vi "pulse_generator_data_v3.vi"(4 "Vapor Inlet Temp [C]":dbl, 5 "Power":dbl, 6 "PG Data":waveform(dbl)[](array[waveform]), 7 "Offsets":T4={"PG Abs"=0.0, "PG Pitot dP"=11500.0, "W1-4 dP "=0.0, "W1-7 dP"=11500.0, "W1-7 Fast dP"=0.0, "TS W1 Abs P"=11500.0, "TS W7 Abs P"=0.0, "Vapor Line Pitot dP"=0.0}, 8 "Session Start Time":timestamp) -> (0 "Pulse Generator Charts":T2, 1 "Diode Charts":T1, 2 "Measurements":T3={"PG Abs Pressure"=119484.80284900061, "Vapor Temperature"=19.805676371442082, "Liquid Temperature"=19.52526901660894, "Tinlet"=121.24568157832624, "Tsectwo"=119.96937909943745, "TS Abs Pressure W1"=121.24568157832624, "TS Abs Pressure W7"=119.96937909943745, "W1-4 dP[Pa]"=19.52526901660894, "W1-7 dP[Pa]"=119.96937909943745, "W1-7 dP[Pa] Fast"=119.96937909943745, "PG Venturi dP [Pa]"=119.96937909943745, "Vapor Line Pitot dP [Pa]"=119.96937909943745, "Tsecthree"=19.191961040039615, "Toutlet"=19.148186089917207, "TS Ext"=18.97439824494449, "Vapor Sat Pressure"=121.24568157832624, "Liquid Sat Pressure"=119.96937909943745, "PG Mass Flow Rate"=nan, "Vapor Line Mass Flow"=119.96937909943745}, 3 "PG Data - Queue":dbl[][](array[numeric]))   [LabVIEW 2017]
uses:
  Sensor Translation/sensor_translation.lvlib
  Sensor Translation/Pressure Transducers/Omega/omega_px209_060a5v.vi
  Sensor Translation/Pressure Transducers/Rosemont/rosemont_3051C_d_1_a_2_2_a_1_a.vi
  Sensor Translation/Pressure Transducers/Omega/omega_px409_2-5ddui.vi
  diode_charts.ctl
  <vilib>/Waveform/WDTOps.llb/WDT Get Waveform Time Array DBL.vi
  pulse_generator_data_controls.ctl
  pulse_generator_data.ctl
  pulse_generator_data_charts.ctl
panel:
  out "Main Diode":dbl[](array[numeric])
  # "Test Section"
  # "Pulse Gen"
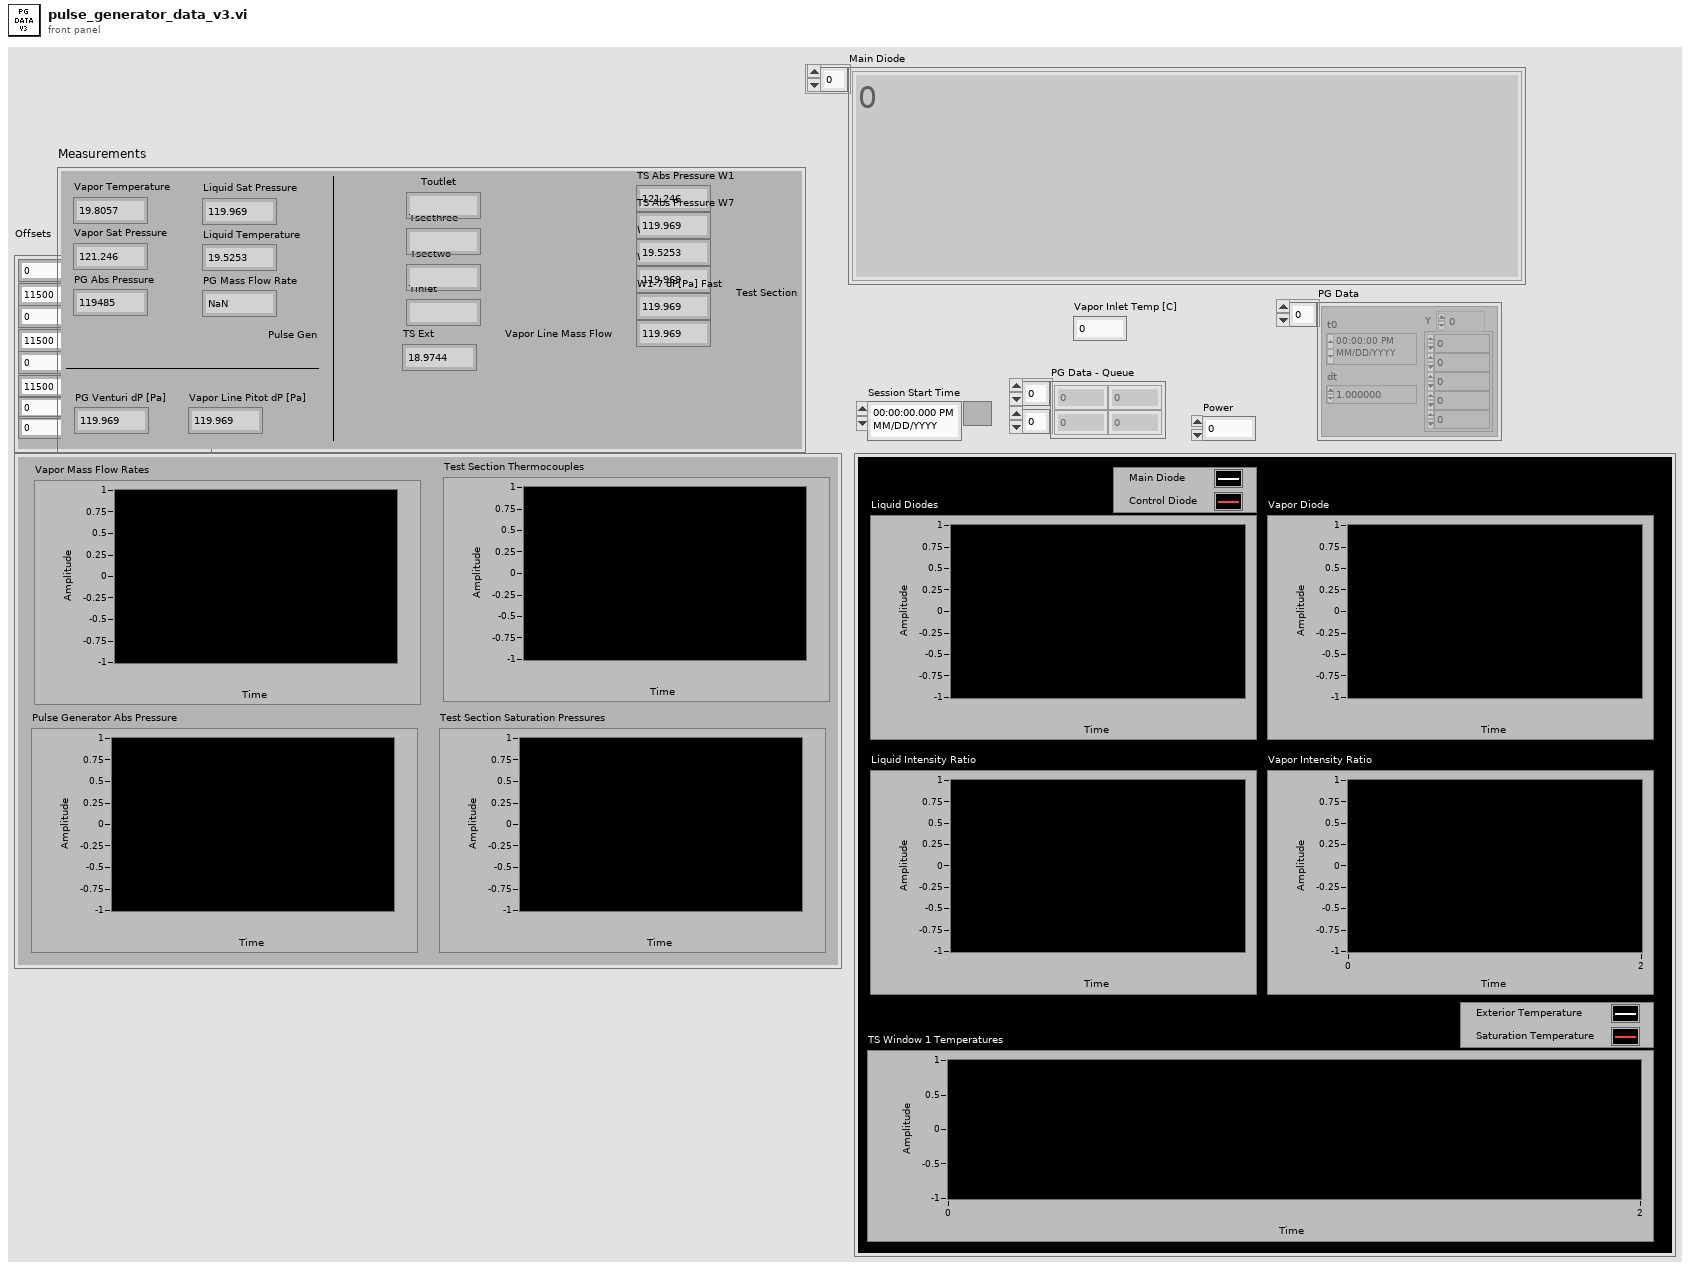
[diagram p1: front panel]
types:
  T1 = typedef "diode_charts.ctl" = cluster{"Liquid Diodes":cluster{dbl, dbl}, "Liquid Intensity Ratio":dbl, "Vapor Diode":cluster{dbl, dbl}, "Vapor Intensity Ratio":dbl, "TS Window 1 Temperatures":cluster{"Average":dbl, "T Sat [C]":dbl}}
  T2 = typedef "pulse_generator_data_charts.ctl" = cluster{"Vapor Mass Flow Rates":cluster{"max value":dbl, "max value":dbl}, "Test Section Thermocouples":cluster{"[0]":dbl, "[1]":dbl, "[2]":dbl, "[3]":dbl, "[4]":dbl}, "Pulse Generator Abs Pressure":dbl[], "Test Section Saturation Pressures":cluster{"max value":dbl, "max value":dbl}}
  T3 = typedef "pulse_generator_data.ctl" = cluster{"PG Abs Pressure":dbl, "Vapor Temperature":dbl, "Liquid Temperature":dbl, "Tinlet":dbl, "Tsectwo":dbl, "TS Abs Pressure W1":dbl, "TS Abs Pressure W7":dbl, "W1-4 dP[Pa]":dbl, "W1-7 dP[Pa]":dbl, "W1-7 dP[Pa] Fast":dbl, "PG Venturi dP [Pa]":dbl, "Vapor Line Pitot dP [Pa]":dbl, "Tsecthree":dbl, "Toutlet":dbl, "TS Ext":dbl, "Vapor Sat Pressure":dbl, "Liquid Sat Pressure":dbl, "PG Mass Flow Rate":dbl, "Vapor Line Mass Flow":dbl}
  T4 = typedef "pulse_generator_data_controls.ctl" = cluster{"PG Abs":dbl, "PG Pitot dP":dbl, "W1-4 dP ":dbl, "W1-7 dP":dbl, "W1-7 Fast dP":dbl, "TS W1 Abs P":dbl, "TS W7 Abs P":dbl, "Vapor Line Pitot dP":dbl}
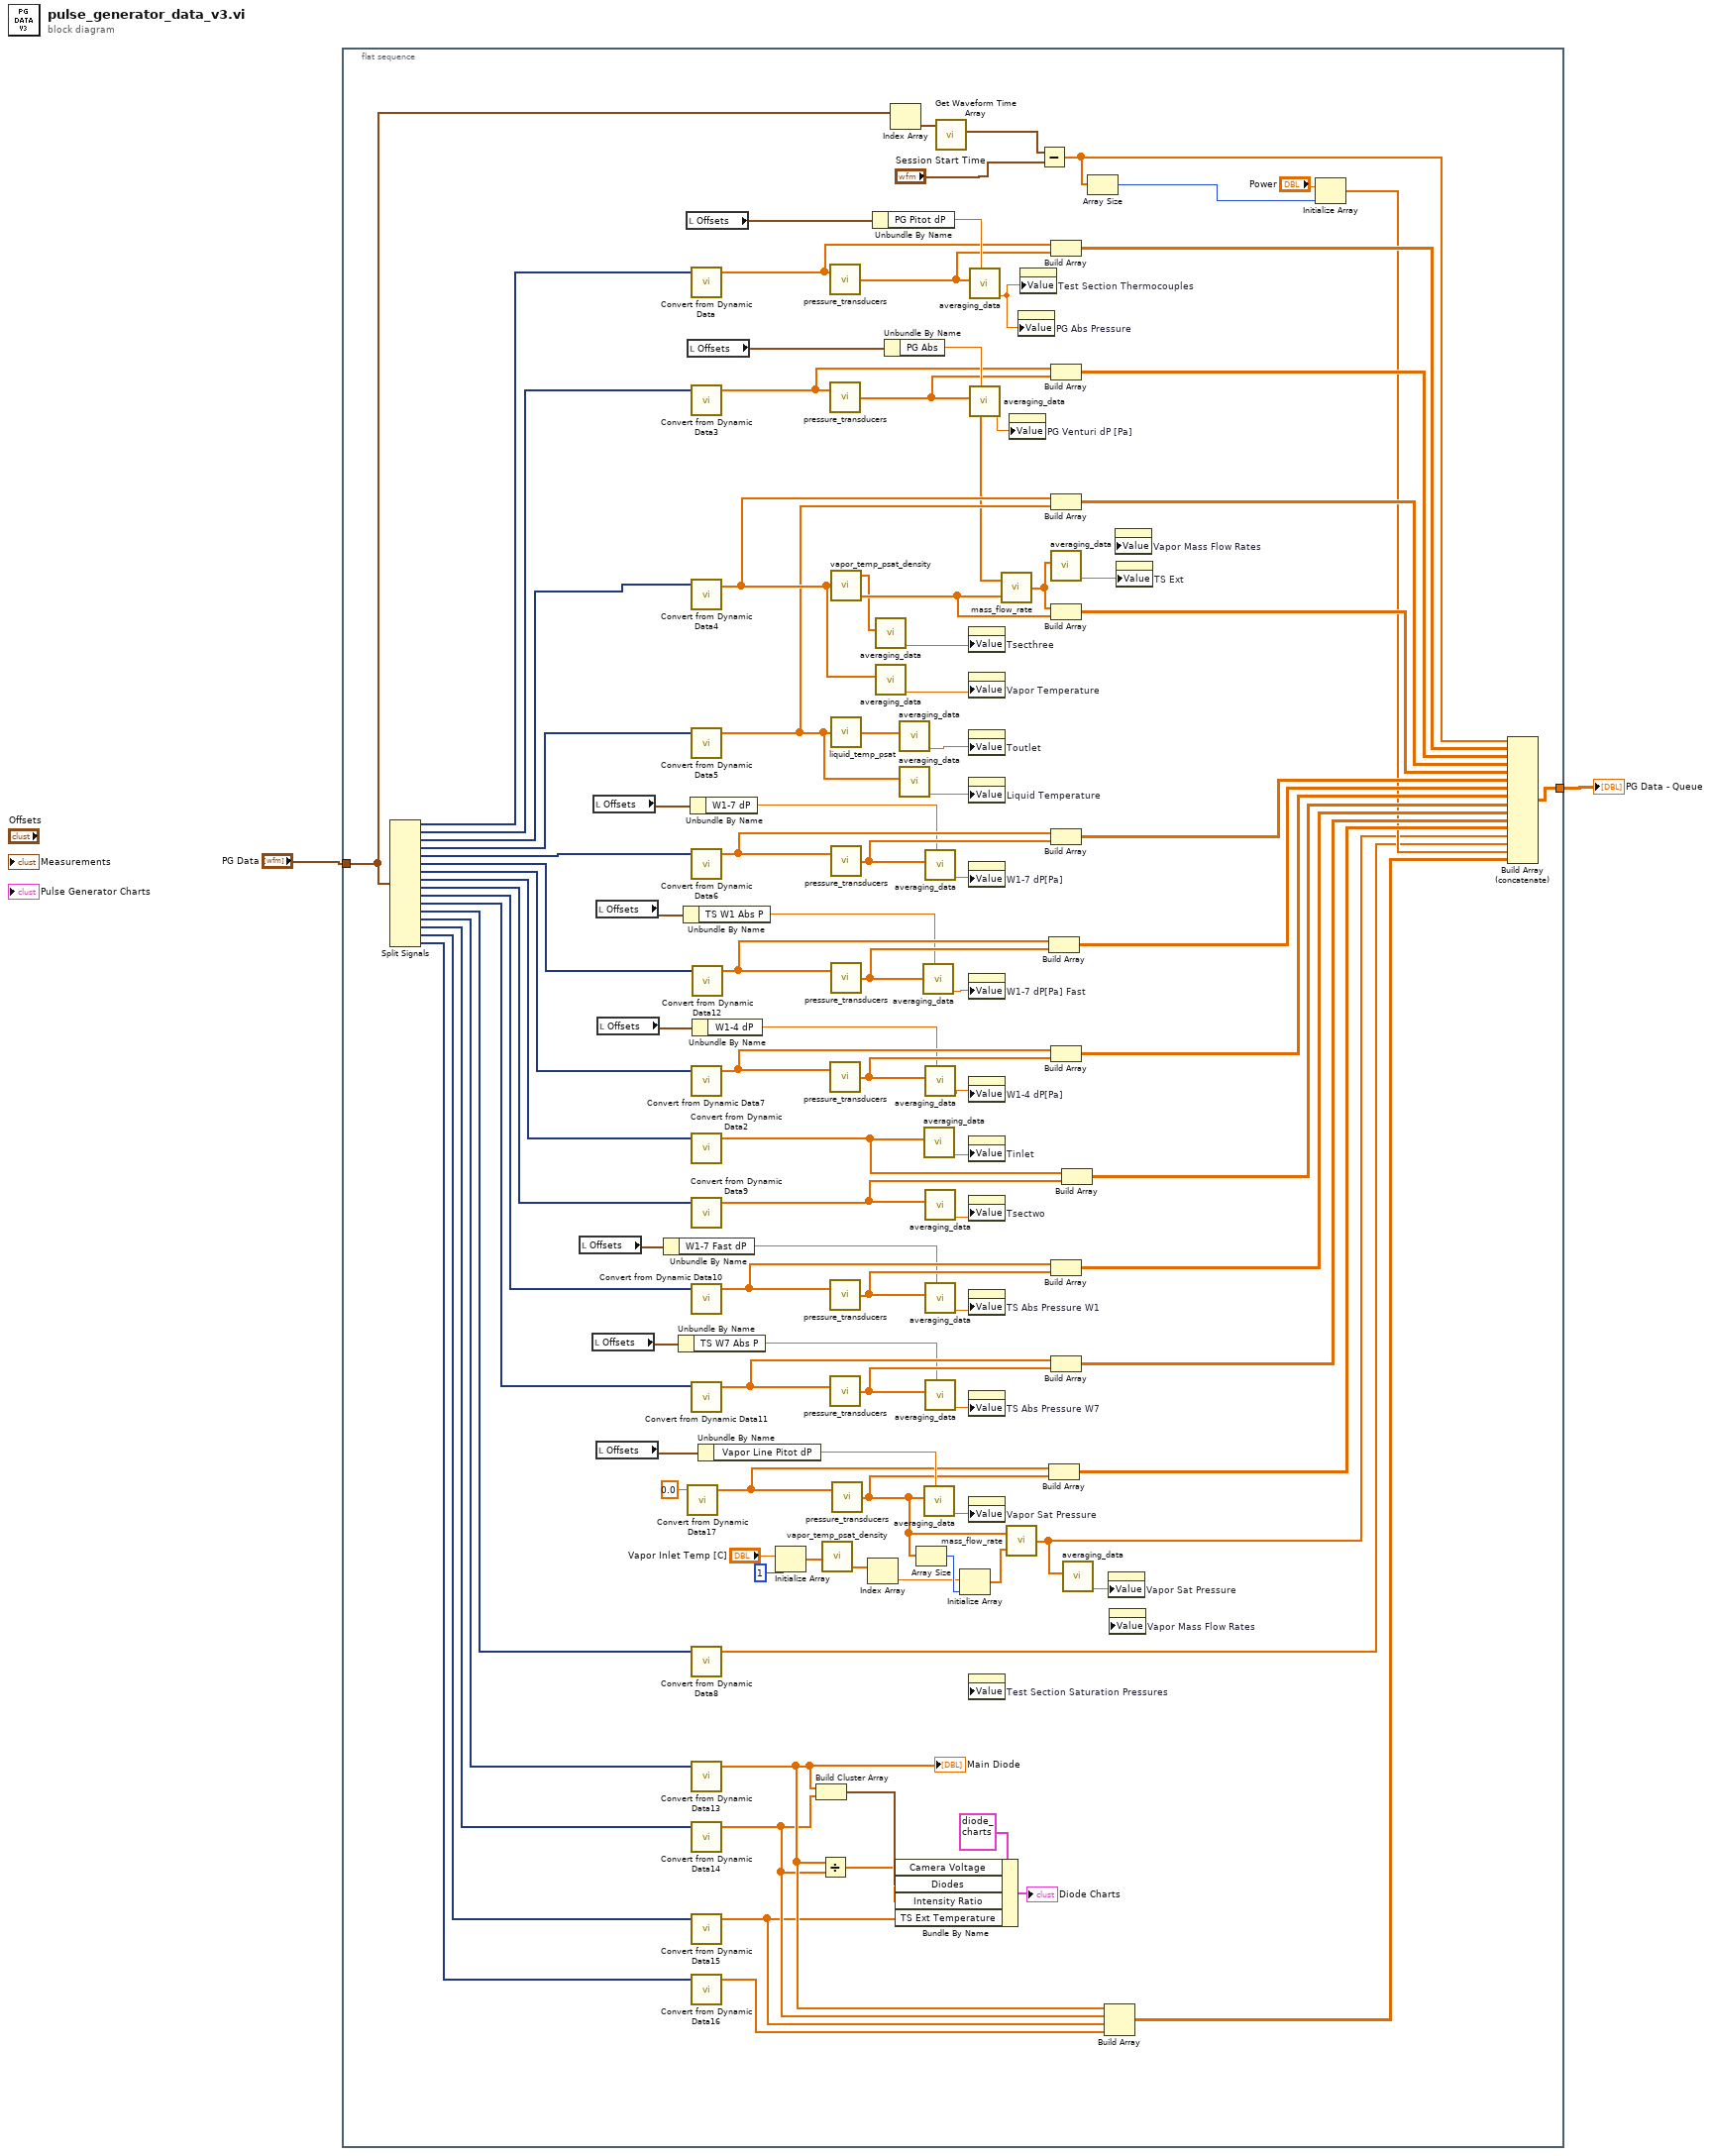
[diagram p0: block diagram]
diagram:
  n1 = flat-sequence {
    tunnel: [w114] -> w2
    tunnel: "PG Data" -> [w105]
    frame #0 {
      n2 = Split Signals(w105) -> (w97:dynamicdata, w110:dynamicdata, w109:dynamicdata, w108:dynamicdata, w107:dynamicdata, w59:dynamicdata, w60:dynamicdata, w61:dynamicdata, w62:dynamicdata, w63:dynamicdata, w64:dynamicdata, w13:dynamicdata, w12:dynamicdata, w11:dynamicdata, w10:dynamicdata, w9:dynamicdata)  [unwired: 16 in]
      n3 = local read "Offsets"() -> (w37:T4)
      n4 = local read "Offsets"() -> (w36:T4)
      n5 = local read "Offsets"() -> (w43:T4)
      n6 = local read "Offsets"() -> (w41:T4)
      n7 = local read "Offsets"() -> (w30:T4)
      n8 = local read "Offsets"() -> (w40:T4)
      n9 = Unbundle By Name(w37) -> ("W1-7 Fast dP"=w33:dbl)
      n10 = Unbundle By Name(w36) -> ("TS W7 Abs P"=w32:dbl)
      n11 = Unbundle By Name(w41) -> ("TS W1 Abs P"=w39:dbl)
      n12 = local read "Offsets"() -> (w104:T4)
      n13 = local read "Offsets"() -> (w102:T4)
      n14 = call "Convert from Dynamic Data17"("Dynamic Data Type"=0.0) -> ("Array"=w27:dbl[])  [unwired: 3 in]
      n15 = Unbundle By Name(w43) -> ("W1-7 dP"=w42:dbl)
      n16 = call "Convert from Dynamic Data"("Dynamic Data Type"=w97) -> ("Array"=w90:dbl[])  [unwired: 3 in]
      n17 = call "Convert from Dynamic Data3"("Dynamic Data Type"=w110) -> ("Array"=w87:dbl[])  [unwired: 3 in]
      n18 = call "Convert from Dynamic Data4"("Dynamic Data Type"=w109) -> ("Array"=w78:dbl[])  [unwired: 3 in]
      n19 = call "Convert from Dynamic Data5"("Dynamic Data Type"=w108) -> ("Array"=w77:dbl[])  [unwired: 3 in]
      n20 = call "Convert from Dynamic Data6"("Dynamic Data Type"=w107) -> ("Array"=w92:dbl[])  [unwired: 3 in]
      n21 = call "Convert from Dynamic Data7"("Dynamic Data Type"=w60) -> ("Array"=w94:dbl[])  [unwired: 3 in]
      n22 = call "Convert from Dynamic Data2"("Dynamic Data Type"=w61) -> ("Array"=w73:dbl[])  [unwired: 3 in]
      n23 = call "Convert from Dynamic Data9"("Dynamic Data Type"=w62) -> ("Array"=w82:dbl[])  [unwired: 3 in]
      n24 = call "Convert from Dynamic Data10"("Dynamic Data Type"=w63) -> ("Array"=w95:dbl[])  [unwired: 3 in]
      n25 = call "Convert from Dynamic Data11"("Dynamic Data Type"=w64) -> ("Array"=w96:dbl[])  [unwired: 3 in]
      n26 = call "Convert from Dynamic Data8"("Dynamic Data Type"=w13) -> ("Array"=w19:dbl[])  [unwired: 3 in]
      n27 = call "Convert from Dynamic Data13"("Dynamic Data Type"=w12) -> ("Array"=w51:dbl[])  [unwired: 3 in]
      "Main Diode" <- w51
      n28 = call "Convert from Dynamic Data14"("Dynamic Data Type"=w11) -> ("Array"=w50:dbl[])  [unwired: 3 in]
      n29 = call "Convert from Dynamic Data15"("Dynamic Data Type"=w10) -> ("Array"=w49:dbl[])  [unwired: 3 in]
      n30 = call "Convert from Dynamic Data16"("Dynamic Data Type"=w9) -> ("Array"=w48:dbl[])  [unwired: 3 in]
      n31 = call "Convert from Dynamic Data12"("Dynamic Data Type"=w59) -> ("Array"=w58:dbl[])  [unwired: 3 in]
      n32 = Unbundle By Name(w40) -> ("W1-4 dP"=w38:dbl)
      n33 = Unbundle By Name(w30) -> ("Vapor Line Pitot dP"=w28:dbl)
      n34 = Initialize Array("Vapor Inlet Temp [C]", 1 ("dimension size")) -> (w15:dbl[])
      n35 = Build Cluster Array(w51, w50) -> (w53:cluster{dbl, dbl}[])
      n36 = Divide(x=w51, y=w50) -> (x/y=w52:dbl[])
      n37 = call "vapor_temp_psat_density.vi"("Vapor Temp [C]"=w15) -> ("Vapor Density"=w14:dbl[])  [unwired: 1 in, 1 out]
      n38 = call-poly "pressure_transducers.vi"("Source"=w90) -> ("Target"=w89:dbl[])  [unwired: 1 in]
      n39 = call-poly "pressure_transducers.vi"("Source"=w87) -> ("Target"=w46:dbl[])  [unwired: 1 in]
      n40 = call-poly "pressure_transducers.vi"("Source"=w94) -> ("Target"=w83:dbl[])  [unwired: 1 in]
      n41 = call-poly "pressure_transducers.vi"("Source"=w95) -> ("Target"=w81:dbl[])  [unwired: 1 in]
      n42 = call-poly "pressure_transducers.vi"("Source"=w96) -> ("Target"=w80:dbl[])  [unwired: 1 in]
      n43 = call "vapor_temp_psat_density.vi"("Vapor Temp [C]"=w78) -> ("Psat Vapor"=w71:dbl[], "Vapor Density"=w79:dbl[])  [unwired: 1 in]
      n44 = call "liquid_temp_psat.vi"("Liquid Temp [C]"=w77) -> ("Psat Liquid"=w65:dbl[])
      n45 = call-poly "pressure_transducers.vi"("Source"=w92) -> ("Target"=w84:dbl[])  [unwired: 1 in]
      n46 = call-poly "pressure_transducers.vi"("Source"=w58) -> ("Target"=w57:dbl[])  [unwired: 1 in]
      n47 = call-poly "pressure_transducers.vi"("Source"=w27) -> ("Target"=w6:dbl[])  [unwired: 1 in]
      n48 = Index Array(array=w14) -> (element=w24:dbl)  [unwired: 1 in]
      n49 = Unbundle By Name(w104) -> ("PG Pitot dP"=w103:dbl)
      n50 = call "averaging_data.vi"("Input"=w71) -> ("Offset Average"=w45:dbl)  [unwired: 6 in, 3 out]
      n51 = call "averaging_data.vi"("Input"=w78) -> ("Offset Average"=w44:dbl)  [unwired: 6 in, 3 out]
      n52 = Unbundle By Name(w102) -> ("PG Abs"=w101:dbl)
      n53 = Index Array(array=w105) -> (element=w106:waveform(dbl))  [unwired: 1 in]
      n54 = Bundle By Name(cluster=T1 {"Liquid Diodes"={0.0, 0.0}, "Liquid Intensity Ratio"=0.0, "Vapor Diode"={0.0, 0.0}, "Vapor Intensity Ratio"=0.0, "TS Window 1 Temperatures"={"Average"=0.0, "T Sat [C]"=0.0}} ("Diode Charts 2"), "Diodes"=w53, "Intensity Ratio"=w52, "TS Ext Temperature"=w49) -> (→"Diode Charts":T1)  [unwired: 1 in]
      n55 = call "averaging_data.vi"("Input"=w65) -> ("Offset Average"=w72:dbl)  [unwired: 6 in, 3 out]
      n56 = call "averaging_data.vi"("Input"=w77) -> ("Offset Average"=w76:dbl)  [unwired: 6 in, 3 out]
      n57 = Array Size(array=w6) -> (size(s)=w25:i32)
      n58 = call "averaging_data.vi"("Offset"=w39, "Input"=w57) -> ("Offset Average"=w35:dbl)  [unwired: 5 in, 3 out]
      n59 = call "averaging_data.vi"("Input"=w73) -> ("Offset Average"=w67:dbl)  [unwired: 6 in, 3 out]
      n60 = call "averaging_data.vi"("Offset"=w28, "Input"=w6) -> ("Offset Average"=w29:dbl)  [unwired: 5 in, 3 out]
      n61 = call "averaging_data.vi"("Offset"=w42, "Input"=w84) -> ("Offset Average"=w75:dbl)  [unwired: 5 in, 3 out]
      n62 = call "averaging_data.vi"("Offset"=w38, "Input"=w83) -> ("Offset Average"=w74:dbl)  [unwired: 5 in, 3 out]
      n63 = call "averaging_data.vi"("Input"=w82) -> ("Offset Average"=w69:dbl)  [unwired: 6 in, 3 out]
      n64 = call "averaging_data.vi"("Offset"=w33, "Input"=w81) -> ("Offset Average"=w68:dbl)  [unwired: 5 in, 3 out]
      n65 = call "averaging_data.vi"("Offset"=w32, "Input"=w80) -> ("Offset Average"=w34:dbl)  [unwired: 5 in, 3 out]
      n66 = call-poly <vilib>:"Get Waveform Time Array.vi"("waveform in"=w106) -> ("X array"=w3:timestamp[])  [unwired: 9 in, 1 out]
      n67 = Initialize Array(w24, w25) -> (w23:dbl[])
      n68 = property on="Tsecthree" class="DigNum (strict)"("Value"=w45) -> ()  [unwired: 2 in, 2 out]
      n69 = property on="Vapor Temperature" class="DigNum (strict)"("Value"=w44) -> ()  [unwired: 2 in, 2 out]
      n70 = property on="Toutlet" class="DigNum (strict)"("Value"=w72) -> ()  [unwired: 2 in, 2 out]
      n71 = property on="Liquid Temperature" class="DigNum (strict)"("Value"=w76) -> ()  [unwired: 2 in, 2 out]
      n72 = property on="W1-7 dP[Pa]" class="DigNum (strict)"("Value"=w75) -> ()  [unwired: 2 in, 2 out]
      n73 = property on="W1-7 dP[Pa] Fast" class="DigNum (strict)"("Value"=w35) -> ()  [unwired: 2 in, 2 out]
      n74 = property on="W1-4 dP[Pa]" class="DigNum (strict)"("Value"=w74) -> ()  [unwired: 2 in, 2 out]
      n75 = property on="Tinlet" class="DigNum (strict)"("Value"=w67) -> ()  [unwired: 2 in, 2 out]
      n76 = property on="Tsectwo" class="DigNum (strict)"("Value"=w69) -> ()  [unwired: 2 in, 2 out]
      n77 = property on="TS Abs Pressure W1" class="DigNum (strict)"("Value"=w68) -> ()  [unwired: 2 in, 2 out]
      n78 = property on="TS Abs Pressure W7" class="DigNum (strict)"("Value"=w34) -> ()  [unwired: 2 in, 2 out]
      n79 = property on="Vapor Sat Pressure" class="DigNum (strict)"("Value"=w29) -> ()  [unwired: 2 in, 2 out]
      n80 = property on="Test Section Saturation Pressures" class="WFChart (strict)" props=["Value"]() -> ()  [unwired: 3 in, 2 out]
      n81 = call "averaging_data.vi"("Offset"=w103, "Input"=w89) -> ("Offset Average"=w7:dbl)  [unwired: 5 in, 3 out]
      n82 = call "averaging_data.vi"("Offset"=w101, "Input"=w46) -> ("Offset Average"=w31:dbl, "Input Offset"=w5:dbl[])  [unwired: 5 in, 2 out]
      n83 = call "mass_flow_rate.vi"("Density"=w79, "dP Pa"=w5) -> ("Mass Flow Rate [g/s] Array"=w70:dbl[])
      n84 = call "mass_flow_rate.vi"("Density"=w23, "dP Pa"=w6) -> ("Mass Flow Rate [g/s] Array"=w18:dbl[])
      n85 = property on="PG Venturi dP [Pa]" class="DigNum (strict)"("Value"=w31) -> ()  [unwired: 2 in, 2 out]
      n86 = property on="PG Abs Pressure" class="DigNum (strict)"("Value"=w7) -> ()  [unwired: 2 in, 2 out]
      n87 = property on="Test Section Thermocouples" class="WFChart (strict)"("Value"=w7) -> ()  [unwired: 2 in, 2 out]
      n88 = Subtract(x=w3, y="Session Start Time") -> (x-y=w99:dbl[])
      n89 = Build Array(w58, w57) -> (w56:dbl[][])
      n90 = Build Array(w27, w6) -> (w26:dbl[][])
      n91 = Build Array(w90, w89) -> (w88:dbl[][])
      n92 = Build Array(w87, w46) -> (w66:dbl[][])
      n93 = Build Array(w78, w77) -> (w86:dbl[][])
      n94 = call "averaging_data.vi"("Input"=w70) -> ("Offset Average"=w47:dbl)  [unwired: 6 in, 3 out]
      n95 = Build Array(w70, w79) -> (w85:dbl[][])
      n96 = Build Array(w92, w84) -> (w91:dbl[][])
      n97 = Build Array(w94, w83) -> (w93:dbl[][])
      n98 = Build Array(w95, w81) -> (w112:dbl[][])
      n99 = Build Array(w96, w80) -> (w111:dbl[][])
      n100 = Build Array(w73, w82) -> (w113:dbl[][])
      n101 = call "averaging_data.vi"("Input"=w18) -> ("Offset Average"=w20:dbl)  [unwired: 6 in, 3 out]
      n102 = Array Size(array=w99) -> (size(s)=w98:i32)
      n103 = Build Array(w51, w50, w49, w48) -> (w22:dbl[][])
      n104 = property on="Vapor Sat Pressure" class="DigNum (strict)"("Value"=w20) -> ()  [unwired: 2 in, 2 out]
      n105 = property on="Vapor Mass Flow Rates" class="WFChart (strict)" props=["Value"]() -> ()  [unwired: 3 in, 2 out]
      n106 = property on="Vapor Mass Flow Rates" class="WFChart (strict)" props=["Value"]() -> ()  [unwired: 3 in, 2 out]
      n107 = property on="TS Ext" class="DigNum (strict)"("Value"=w47) -> ()  [unwired: 2 in, 2 out]
      n108 = Initialize Array("Power", w98) -> (w21:dbl[])
      n109 = Build Array (concatenate)(w99, w88, w66, w86, w85, w91, w56, w93, w113, w112, w111, w26, w18, w19, w21, w22) -> (w114:dbl[][])
    }
  }
  "PG Data - Queue" <- w2
